vi "Rotation3d_GetAxisAngle.vi"(11 "in Rotation3d":T1={"Q_quaternion"={"R"=1.0, "V"=[0.0, 0.0, 0.0]}}) -> (1 "Angle":dbl, 3 "Axis Vector":dbl[](array[numeric]))   [LabVIEW 2019, in "Trajectory_Library.lvlib"]
doc: "Returns the axis in the axis-angle representation of this rotation and the angle in radians in the axis-angle representation of this rotation.\n\nParameters:\n - in ROTATION3D - This ROTATION3D data structure\n\nReturns:\n - Axis -- The axis in the axis-angle representation.\n - Angle -- The angle in radians in the axis-angle representation of this rotation"
uses:
  Trajectory_Library.lvlib
  TypeDef/QUATERNION.ctl
  TypeDef/ROTATION3D.ctl
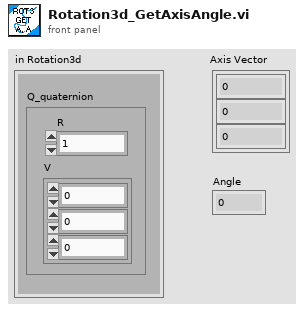
[diagram p1: front panel]
types:
  T1 = typedef "Trajectory_Library.lvlib/ROTATION3D.ctl" = cluster{"Q_quaternion":T2}
  T2 = typedef "Trajectory_Library.lvlib/QUATERNION.ctl" = cluster{"R":dbl, "V":dbl[]}
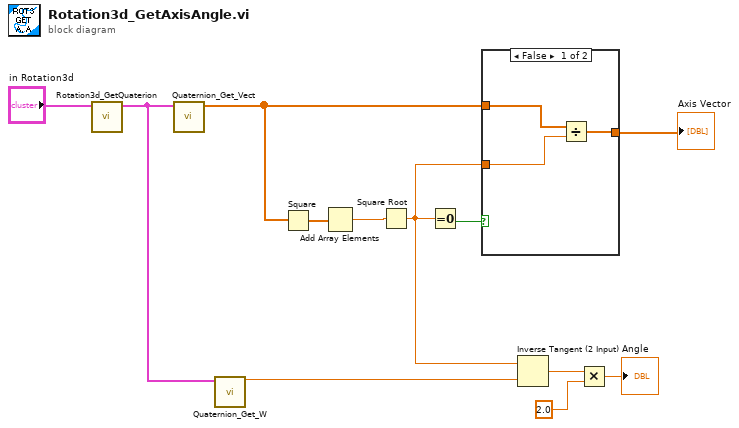
[diagram p0: block diagram]
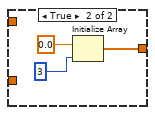
[diagram p2: hidden frame]
diagram:
  n1 = call "Rotation3d_GetQuaterion.vi"("in Rotation3d"="in Rotation3d") -> ("out Quaterion"=w5:T2)  [unwired: 10 in]
  n2 = call "Quaternion_Get_Vect.vi"("Quaternion"=w5) -> ("Vector"=w7:dbl[])  [unwired: 10 in]
  n3 = call "Quaternion_Get_W.vi"("Quaternion"=w5) -> ("W"=w4:dbl)  [unwired: 10 in]
  n4 = Square(x=w7) -> (x^2=w9:dbl[])
  n5 = Add Array Elements(numeric array=w9) -> (sum=w8:dbl)
  n6 = Square Root(x=w8) -> (sqrt(x)=w6:dbl)
  n7 = Equal To 0?(x=w6) -> (x = 0?=w11:bool)
  n8 = case shown="False" w11 {
    tunnel: [w13 w16] -> w10
    tunnel: w7 -> [w15 _]
    tunnel: w6 -> [w14 _]
    frame False {
      n9 = Divide(x=w15, y=w14) -> (x/y=w13:dbl[])
    }
    frame True {
      n10 = Initialize Array(0.0 ("element"), 3 ("dimension size")) -> (w16:dbl[])
    }
  }
  "Axis Vector" <- w10
  n11 = Inverse Tangent (2 Input)(1:w4, 2:w6) -> (0:w3:dbl)
  n12 = Multiply(x=w3, y=2.0) -> (x*y=→"Angle":dbl)
